vi "MotorOutputs.vi"(7 "Max Wheel Speed":dbl, 8 "error in (no error)":errorcluster, 9 "Motor Speeds":dbl[](array[numeric]), 10 "Target Angles":dbl[](array[numeric]), 11 "Steering Refnums In":T8) -> (0 "error out":errorcluster, 1 "Speed Motor Setpoints":dbl[](array[numeric]), 2 "Steering Motor Setpoints":dbl[](array[numeric]), 3 "Steering Refnums Out":T8)   [LabVIEW 2015, in "Team900SwerveDrive.lvlib"]
uses:
  Team900SwerveDrive.lvlib
  <vilib>/Rock Robotics/WPI/MotorControl/WPI_MotorControlDeviceRef.ctl
  <vilib>/Rock Robotics/WPI/MotorControl/WPI_MotorControlType.ctl
  <vilib>/Rock Robotics/SystemInterfaces/DIO/FPGA_DIOPWMChannel.ctl
  <vilib>/Rock Robotics/WPI/PWM/WPI_PWMDeadband.ctl
  <vilib>/Rock Robotics/WPI/CAN/Jaguar/SubVIs/WPI_CANJaguar_ControlMode.ctl
  <vilib>/Rock Robotics/WPI/CAN/TalonSRX/WPI_CANTalonSRX_APIControlMode.ctl
  SwerveGlobalData.vi
panel:
  out "Speed Cluster":T9 {"RR Speed" scale=-1.0..1.0; "RL Speed" scale=-1.0..1.0; "FR Speed" scale=-1.0..1.0; "FL Speed" scale=-1.0..1.0}
  out "Angle Cluster":T10 {"FL Angle" scale=3.1416..-3.1416; "FR Angle" scale=3.1416..-3.1416; "RR Angle" scale=3.1416..-3.1416; "RL Angle" scale=3.1416..-3.1416}
  # "This VI takes the target angles (in radians) and the target\nspeeds (from 0 to 1, in units of proportion of max speed)\nand converts them to setpoints for the steering and speed\nTalon SRX's."
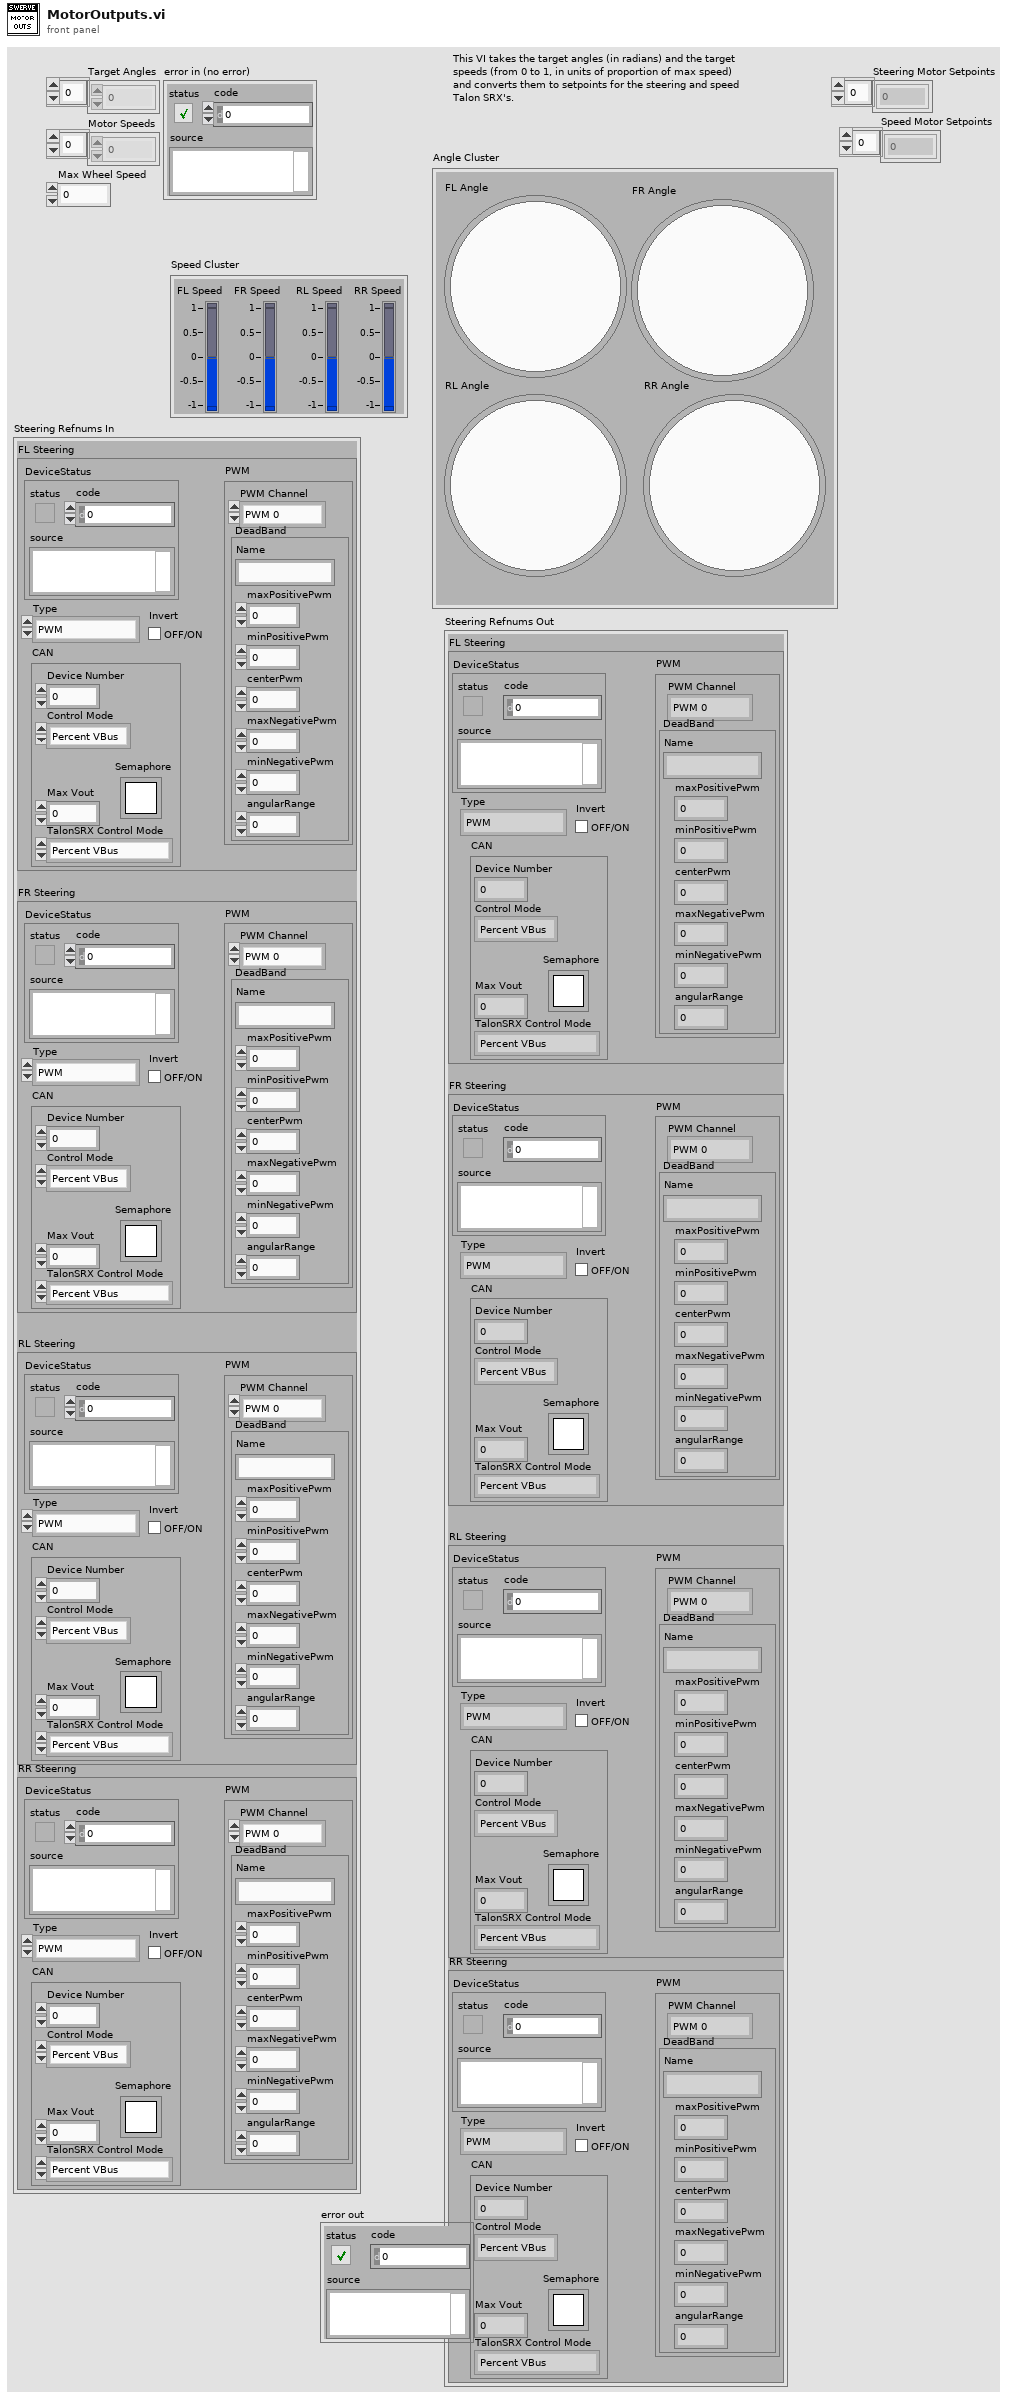
[diagram p1: front panel]
types:
  T1 = typedef "WPI_MotorControlDeviceRef.ctl" = cluster{"DeviceStatus":errorcluster, "Type":T2, "PWM":cluster{"PWM Channel":T3, "DeadBand":T4}, "CAN":cluster{"Device Number":u8, "Control Mode":T5, "Semaphore":T6, "Max Vout":dbl, "TalonSRX Control Mode":T7}, "Invert":bool}
  T2 = typedef "WPI_MotorControlType.ctl" = enum16{"PWM", "CAN", "CANTalonSRX"}
  T3 = typedef "FPGA_DIOPWMChannel.ctl" = enum8{"PWM 0", "PWM 1", "PWM 2", "PWM 3", "PWM 4", "PWM 5", "PWM 6", "PWM 7", "PWM 8", "PWM 9", "PWM MXP 0", "PWM MXP 1", "PWM MXP 2", "PWM MXP 3", "PWM MXP 4", "PWM MXP 5", "PWM MXP 6", "PWM MXP 7", "PWM MXP 8", "PWM MXP 9", "Invalid"}
  T4 = typedef "WPI_PWMDeadband.ctl" = cluster{"Name":string, "maxPositivePwm":i32, "minPositivePwm":i32, "centerPwm":i32, "maxNegativePwm":i32, "minNegativePwm":i32, "angularRange":u16}
  T5 = typedef "WPI_CANJaguar_ControlMode.ctl" = enum8{"Percent VBus", "Current", "Speed", "Position", "Voltage"}
  T6 = typedef "Semaphore RefNum" = refnum<k1>
  T7 = typedef "WPI_CANTalonSRX_APIControlMode.ctl" = enum8{"Percent VBus", "Speed", "Position", "Slave", "Unchanged / Invalid", "Voltage Compensation", "Current", "Motion Profile"}
  T8 = cluster{"FL Steering":T1, "FR Steering":T1, "RL Steering":T1, "RR Steering":T1}
  T9 = cluster{"FL Speed":dbl, "FR Speed":dbl, "RL Speed":dbl, "RR Speed":dbl}
  T10 = cluster{"FL Angle":dbl, "FR Angle":dbl, "RL Angle":dbl, "RR Angle":dbl}
  T11 = cluster{"[0]":dbl, "[1]":dbl, "[2]":dbl, "[3]":dbl}
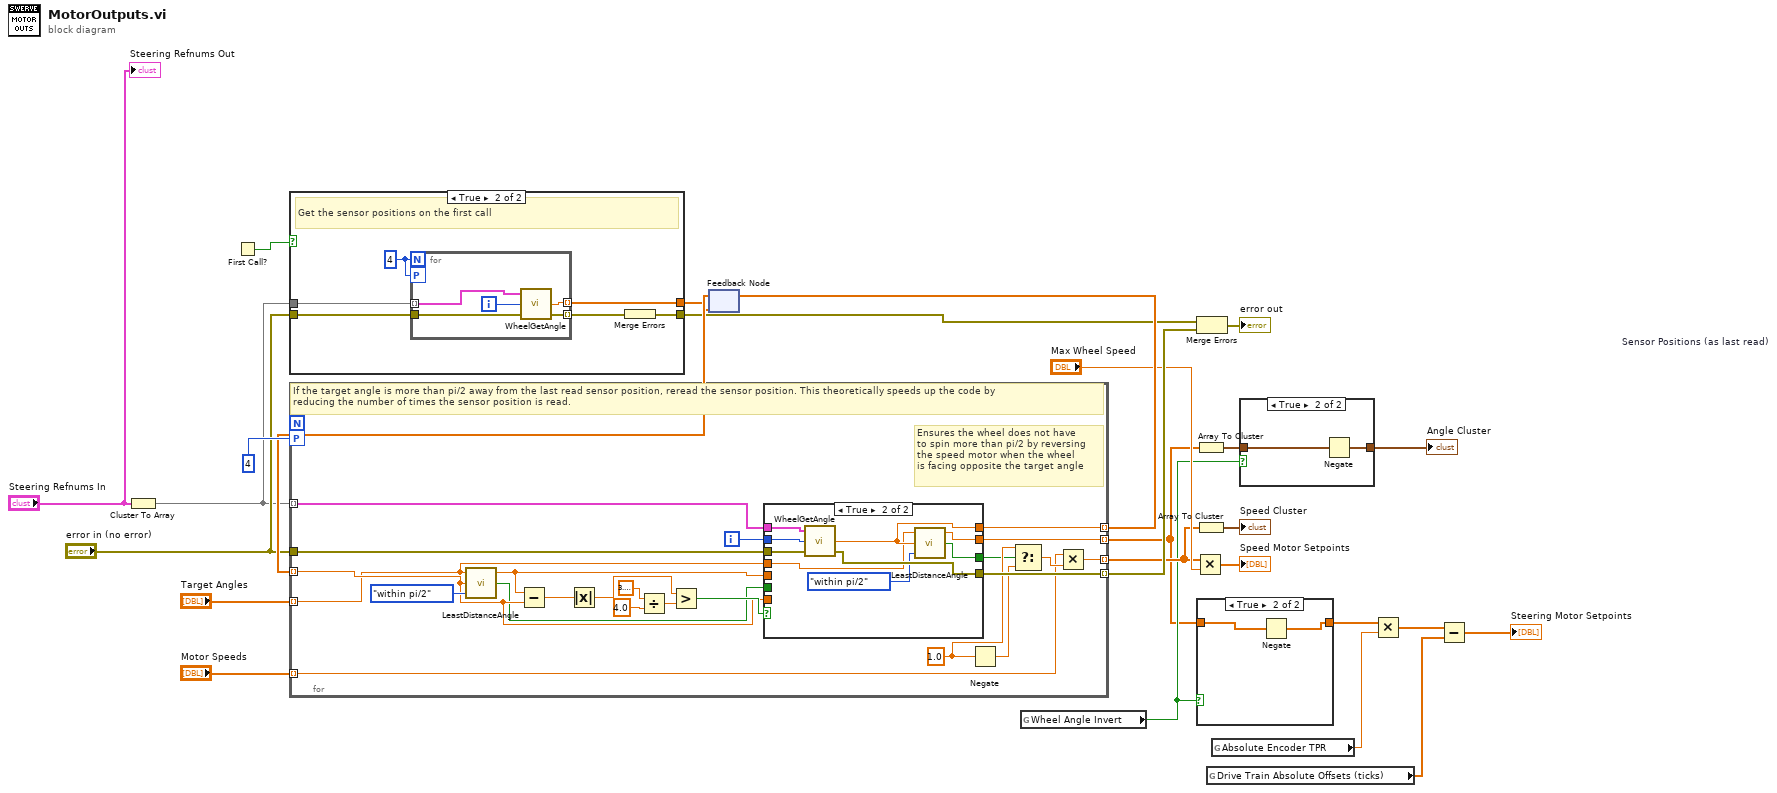
[diagram p0: block diagram]
diagram:
  w26 = 4
  n1 = Cluster To Array(cluster="Steering Refnums In") -> (array=w4:T1[])
  n2 = First Call?() -> (First Call?: T/F=w23:bool)
  n3 = case shown="True" w23 {
    tunnel: "error in (no error)" -> [w27 w33]
    tunnel: [w27 w32] -> w22
    tunnel: w4 -> [_ w31]
    tunnel: [_ w30] -> w17
    frame False {
    }
    frame True {
      w28 = 4
      # "Get the sensor positions on the first call"
      n4 = for {
        N: w28 -> [_]
        tunnel: [w37] -> w30 mode=indexing
        tunnel: w33 -> [w38]
        tunnel: [w36] -> w29 mode=indexing
        workers-P: w28 -> [_]
        tunnel: w31 -> [w35] mode=indexing
        i -> [w34]
        n5 = call "WheelGetAngle.vi"("error in (no error)"=w38, "Wheel"=w34, "CAN Talon SRX Ref"=w35) -> ("error out"=w36:errorcluster, "Sensor Position (rad)"=w37:dbl)  [unwired: 1 out]
      }
      n6 = Merge Errors(w29) -> (w32:errorcluster)
    }
  }
  n7 = feedback #1 "Sensor Positions (as last read)"(w17) -> (w24:dbl[])
  n8 = for {
    N: w26 -> [_]
    workers-P: w26 -> [_]
    tunnel: [w61] -> w25 mode=indexing
    tunnel: "Target Angles" -> [w39] mode=indexing
    tunnel: w24 -> [w50] mode=indexing
    tunnel: "error in (no error)" -> [w60]
    tunnel: [w59] -> w19 mode=indexing
    tunnel: w4 -> [w57] mode=indexing
    tunnel: "Motor Speeds" -> [w45] mode=indexing
    tunnel: [w44] -> w12 mode=indexing
    tunnel: [w42] -> w2 mode=indexing
    i -> [w56]
    w48 = 1.0 ("t")
    # "Ensures the wheel does not have\nto spin more than pi/2 by reversing\nthe speed motor when the wheel\nis facing opposite the target angle"
    # "If the target angle is more than pi/2 away from the last read sensor position, reread the sensor position. This theoretically speeds up the code by\nreducing the number of times the sensor position is read."
    n9 = call "LeastDistanceAngle.vi"("Enum"=enum16{"within pi", "within pi/2"}."within pi/2", "Current angle"=w50, "target angle (between pi and -pi) 2"=w39) -> ("Reverse?"=w40:bool, "output angle"=w43:dbl)  [unwired: 1 out]
    n10 = Subtract(x=w43, y=w50) -> (x-y=w49:dbl)
    n11 = Absolute Value(x=w49) -> (abs(x)=w55:dbl)
    n12 = Divide(x=3.141592653589793, y=4.0) -> (x/y=w52:dbl)
    n13 = Greater?(x=w55, y=w52) -> (0:w58:bool)
    n14 = case shown="True" w58 {
      tunnel: [w65 w69] -> w61
      tunnel: w50 -> [w65 _]
      tunnel: w60 -> [w64 w72]
      tunnel: [w64 w71] -> w59
      tunnel: w57 -> [_ w74]
      tunnel: w56 -> [_ w73]
      tunnel: w43 -> [w63 _]
      tunnel: [w63 w66] -> w42
      tunnel: [w62 w67] -> w41
      tunnel: w40 -> [w62 _]
      tunnel: w39 -> [_ w68]
      frame False {
      }
      frame True {
        n15 = call "WheelGetAngle.vi"("error in (no error)"=w72, "Wheel"=w73, "CAN Talon SRX Ref"=w74) -> ("error out"=w71:errorcluster, "Sensor Position (rad)"=w69:dbl)  [unwired: 1 out]
        n16 = call "LeastDistanceAngle.vi"("Enum"=enum16{"within pi", "within pi/2"}."within pi/2", "Current angle"=w69, "target angle (between pi and -pi) 2"=w68) -> ("Reverse?"=w67:bool, "output angle"=w66:dbl)  [unwired: 1 out]
      }
    }
    n17 = Negate(x=w48) -> (-x=w47:dbl)
    n18 = Select(t=w48, s=w41, f=w47) -> (s? t:f=w46:dbl)
    n19 = Multiply(x=w45, y=w46) -> (x*y=w44:dbl)
  }
  n20 = feedback-in #1(w25) -> ()
  n21 = global read "SwerveGlobalData.vi" "Wheel Angle Invert"() -> (w5:bool)
  n22 = Multiply(x=w12, y="Max Wheel Speed") -> (x*y=→"Speed Motor Setpoints":dbl[])
  n23 = Array To Cluster(array=w2) -> (cluster=w6:T11)
  n24 = Array To Cluster(array=w12) -> (cluster=→"Speed Cluster":T11)
  n25 = Merge Errors(w22, w19) -> (→"error out":errorcluster)
  n26 = case shown="True" w5 {
    tunnel: w2 -> [w75 w77]
    tunnel: [w75 w76] -> w1
    frame False {
    }
    frame True {
      n27 = Negate(x=w77) -> (-x=w76:dbl[])
    }
  }
  n28 = global read "SwerveGlobalData.vi" "Drive Train Absolute Offsets (ticks)"() -> (w9:dbl[])
  n29 = global read "SwerveGlobalData.vi" "Absolute Encoder TPR"() -> (w11:dbl)
  n30 = case shown="True" w5 {
    tunnel: w6 -> [w78 w80]
    tunnel: [w78 w79] -> w7
    frame False {
    }
    frame True {
      n31 = Negate(x=w80) -> (-x=w79:T11)
    }
  }
  "Angle Cluster" <- w7
  n32 = Multiply(x=w1, y=w11) -> (x*y=w8:dbl[])
  n33 = Subtract(x=w8, y=w9) -> (x-y=→"Steering Motor Setpoints":dbl[])
  "Steering Refnums Out" <- "Steering Refnums In"
